vi "AxisGoHome.vi"(8 "error in (no error)":errorcluster, 11 "DMC 3600 in":refnum<class "DMC 3600.lvclass">) -> (0 "error out":errorcluster, 3 "DMC 3600 out":refnum<class "DMC 3600.lvclass">)   [LabVIEW 2019, in "DMC 3600.lvclass"]
uses:
  DMC 3600.lvclass
  LLB/DMC3600/LTDMC.lvlib
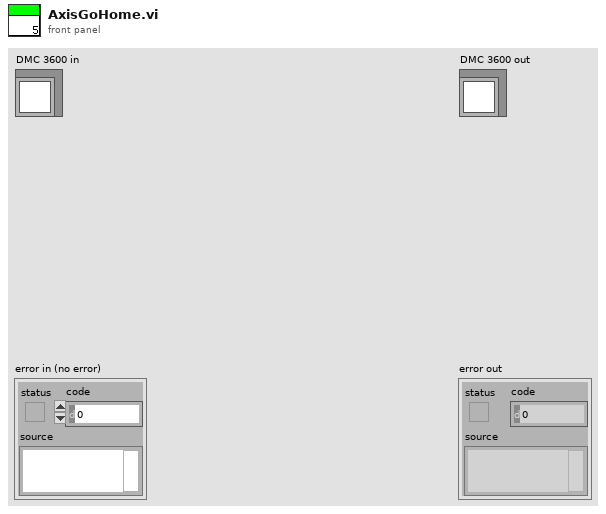
[diagram p1: front panel]
types:
  T1 = cluster{"AxisName":string, "Accel":dbl, "Deaccel":dbl, "Speed":dbl, "Sramp":dbl}[]
  T2 = cluster{"AxisName":string, "Accel":dbl, "Deaccel":dbl, "Speed":dbl, "Sramp":dbl}
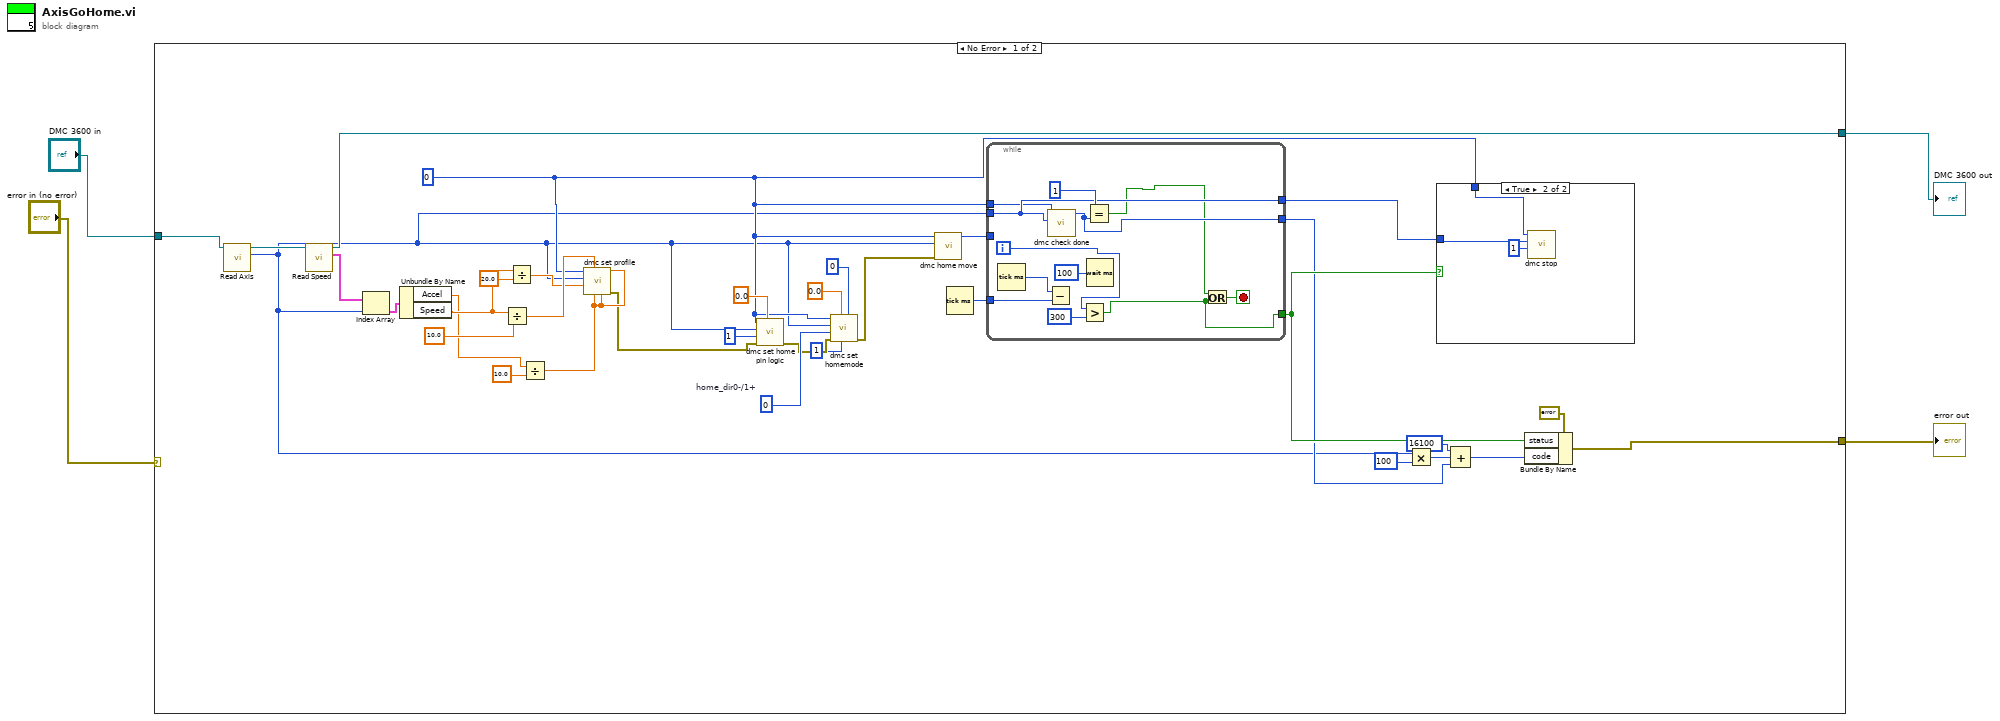
[diagram p0: block diagram]
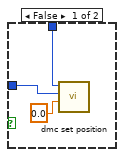
[diagram p2: hidden frame]
diagram:
  n1 = case shown="No Error" "error in (no error)" {
    selector: "error in (no error)" -> [_ w58]
    tunnel: "DMC 3600 in" -> [w23 w59]
    tunnel: [w17 w58] -> w2
    tunnel: [w16 w59] -> w1
    frame No Error {
      w13 = u16 0  # home_dir0-/1+
      w8 = u16 0 ("CardNo")
      n2 = call-dynamic "Read Axis.vi"("AxisCard in"=w23) -> ("Axis"=w6:u32, "AxisCard out"=w39:refnum<class "DMC 3600.lvclass">)  [unwired: 8 in, 1 out]
      n3 = call-dynamic "Read Speed.vi"("AxisCard in"=w39) -> ("AxisSpeed"=w38:T1, "AxisCard out"=w16:refnum<class "DMC 3600.lvclass">)  [unwired: 8 in, 1 out]
      n4 = Index Array(array=w38, index=w6) -> (element=w37:T2)
      n5 = Unbundle By Name(w37) -> ("Accel"=w19:dbl, "Speed"=w35:dbl)
      n6 = Divide(x=w35, y=10.0) -> (x/y=w22:dbl)
      n7 = Divide(x=w35, y=20.0) -> (x/y=w21:dbl)
      n8 = Divide(x=w19, y=10.0) -> (x/y=w18:dbl)
      n9 = call "dmc set profile.vi"("stop_vel"=w18, "Tdec"=w18, "Tacc"=w18, "Max_Vel"=w22, "Min_Vel"=w21, "axis"=w6, "CardNo"=w8) -> ("error out"=w7:errorcluster)  [unwired: 3 in, 1 out]
      n10 = call "dmc set home pin logic.vi"("filter"=0.0, "error in (no error)"=w7, "org_logic"=u16 1, "axis"=w6, "CardNo"=w8) -> ("error out"=w12:errorcluster)  [unwired: 5 in, 1 out]
      n11 = call "dmc set homemode.vi"("EZ_count"=u16 0, "mode"=u16 1, "vel"=0.0, "error in (no error)"=w12, "home_dir"=w13, "axis"=w6, "CardNo"=w8) -> ("error out"=w5:errorcluster)  [unwired: 3 in, 1 out]
      n12 = call "dmc home move.vi"("error in (no error)"=w5, "axis"=w6, "CardNo"=w8) -> ("function return"=w32:i16)  [unwired: 7 in, 1 out]
      n13 = Tick Count (ms)() -> (millisecond timer value=w33:u32)
      n14 = while {
        tunnel: w6 -> [w49]
        tunnel: w33 -> [w55]
        tunnel: w32 -> [_]
        tunnel: [w49] -> w31
        tunnel: [w46] -> w25
        tunnel: [w50] -> w24
        tunnel: w8 -> [w48]
        i -> [w51]
        stop <- w53 stop-if-true
        n15 = Tick Count (ms)() -> (millisecond timer value=w56:u32)
        n16 = Subtract(x=w56, y=w55) -> ()  [unwired: 1 out]
        n17 = call "dmc check done.vi"("axis"=w49, "CardNo"=w48) -> ("function return"=w50:i16)  [unwired: 8 in, 1 out]
        n18 = Greater?(x=w51, y=u32 300) -> (0:w46:bool)
        n19 = Equal?(x=u32 1, y=w50) -> (x = y?=w47:bool)
        n20 = Wait (ms)(milliseconds to wait=u32 100) -> ()  [unwired: 1 out]
        n21 = Or(x=w47, y=w46) -> (x .or. y?=w53:bool)
      }
      n22 = Multiply(x=w6, y=u32 100) -> (x*y=w29:u32)
      n23 = case shown="True" w25 {
        tunnel: w31 -> [w42 w44]
        tunnel: w8 -> [w40 w45]
        frame False {
          n24 = call "dmc set position.vi"("current_position"=0.0 ("Pos"), "axis"=w42, "CardNo"=w40) -> ()  [unwired: 7 in, 2 out]
        }
        frame True {
          n25 = call "dmc stop.vi"("stop_mode"=u16 1, "axis"=w44, "CardNo"=w45) -> ()  [unwired: 7 in, 2 out]
        }
      }
      n26 = Compound Arithmetic op=ADD(16100, w29, w24) -> (w26:u32)
      n27 = Bundle By Name(cluster=errorcluster {"status"=FALSE, "code"=0, "source"=""} ("error constant"), "status"=w25, "code"=w26) -> (w17:errorcluster)
    }
    frame Error {
    }
  }
  "error out" <- w2
  "DMC 3600 out" <- w1
